vi "write full file.vi"(8 "error in":errorcluster, 10 "strings":string, 11 "file path":path) -> (0 "error out":errorcluster)   [LabVIEW 2013, in "NISE_CEF_TreeSerializer.lvlib"]
doc: "Writes the full binary contents of a file."
uses:
  NISE_CEF_TreeSerializer.lvlib
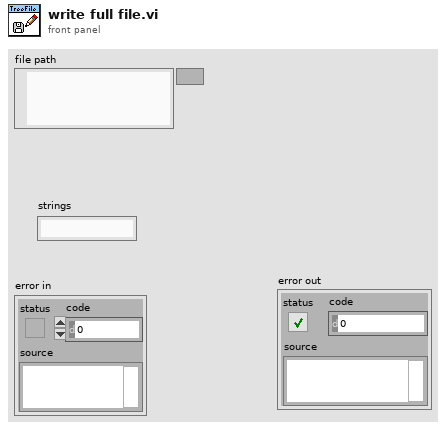
[diagram p1: front panel]
types:
  T1 = enum16{"open", "replace", "create", "open or create", "replace or create", "replace or create with confirmation"}
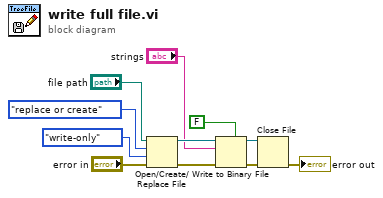
[diagram p0: block diagram]
diagram:
  n1 = Open/Create/Replace File(file path (use dialog)="file path", error in="error in", operation (0:open)=T1."replace or create", access (0:read/write)=enum16{"read/write", "read-only", "write-only"}."write-only") -> (refnum out=w7:refnum<file>, error out=w6:errorcluster)  [unwired: 2 in, 1 out]
  n2 = Write to Binary File(file (use dialog)=w7, data="strings", error in=w6, 5:FALSE ("prepend array or string size? (T)")) -> (refnum out=w11:refnum<file>, error out=w10:errorcluster)  [unwired: 2 in, 1 out]
  n3 = Close File(refnum=w11, error in=w10) -> (error out=→"error out":errorcluster)  [unwired: 1 out]
